vi "Get_Next_Sub_Collection.vi"(8 "error in (no error)":errorcluster caption="entrée d'erreur (pas d'erreur)", 11 "Firebase Packaging en entrée":refnum<class "Firebase Packaging.lvclass">) -> (0 "error out":errorcluster caption="sortie d'erreur", 3 "Firebase Packaging en sortie":refnum<class "Firebase Packaging.lvclass">)   [LabVIEW 2020, in "Library Instrument & Equipement.lvlib" / "Library FireBase.lvlib" / "Firebase Packaging.lvclass"]
doc: "Return the documents present in the test collection for each DATA read with Get_Data\nPlease initialise the following values\n - Name BDD\n - Document of test sequence\n - API Key\n - Nb To Read"
uses:
  Firebase Packaging.lvclass
  C:/Users/ngarcin/OneDrive - Altyor/Standard TB/Class/Firebase/Source/Firebase Driver/Firebase Driver.lvclass
  Firebase Packaging.lvclass/Firebase Packaging.ctl
  JSON API/JSON Value/JSON Value.lvclass
  JSON API/JSON Value/Set from JSON string.vi
  Firebase Altyor/Firebase Altyor.lvclass
  JSON API/Variant JSON/Variant JSON.lvlib
  JSON API/Get Polymorphic/JSON GetSet.lvlib
  Firebase Driver/Firebase Driver.lvclass
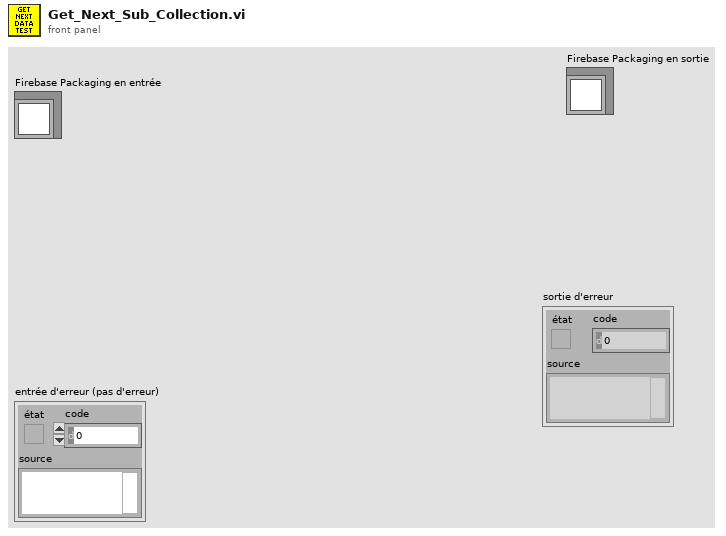
[diagram p1: front panel]
types:
  T1 = cluster{"documents":cluster{"name":string, "fields":cluster{"Result":cluster{"booleanValue":bool}, "CreationDate":cluster{"timestampValue":string}, "Batch":cluster{"stringValue":string}, "SerialNumber":cluster{"stringValue":string}, "EndOfProduction":cluster{"timestampValue":string}, "PartNumber":cluster{"stringValue":string}, "OrderNumber":cluster{"stringValue":string}, "Operator":cluster{"stringValue":string}}}[]}
  T2 = cluster{"name":string, "fields":cluster{"SN_Produit":cluster{"stringValue":string}, "Product_Name":cluster{"stringValue":string}}}[][]
  T3 = cluster{"name":string, "fields":cluster{"Result":cluster{"booleanValue":bool}, "CreationDate":cluster{"timestampValue":string}, "Batch":cluster{"stringValue":string}, "SerialNumber":cluster{"stringValue":string}, "EndOfProduction":cluster{"timestampValue":string}, "PartNumber":cluster{"stringValue":string}, "OrderNumber":cluster{"stringValue":string}, "Operator":cluster{"stringValue":string}}}[]
  T4 = cluster{"name":string, "fields":cluster{"SN_Produit":cluster{"stringValue":string}, "Product_Name":cluster{"stringValue":string}}}[]
  T5 = cluster{"documents":cluster{"name":string, "fields":cluster{"SN_Produit":cluster{"stringValue":string}, "Product_Name":cluster{"stringValue":string}}}[], "nextPageToken":string}
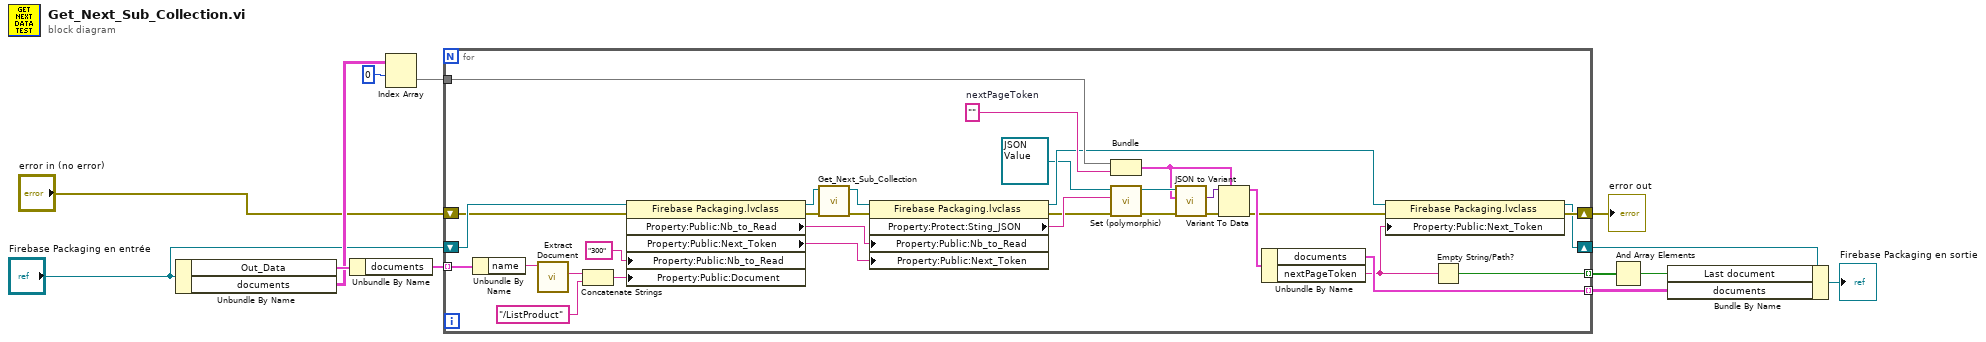
[diagram p0: block diagram]
diagram:
  n1 = Unbundle By Name("Firebase Packaging en entrée") -> ("Out_Data"=w13:T1, "documents"=w10:T2)
  n2 = Unbundle By Name(w13) -> ("documents"=w12:T3)
  n3 = Index Array(array=w10, index (row)=0 ("indice (ligne)")) -> (element=w9:T4)  [unwired: 1 in]
  n4 = for {
    tunnel: [w21] -> w11 mode=indexing
    shift-right: [w23] -> w7
    shift-left: "Firebase Packaging en entrée" -> [w38]
    shift-right: [w25] -> w3
    shift-left: "error in (no error)" -> [w37]
    tunnel: w12 -> [w36] mode=indexing
    tunnel: w9 -> [w28]
    tunnel: [w14] -> w2 mode=indexing
    w40 = ""  # nextPageToken
    n5 = Unbundle By Name(w36) -> ("name"=w35:string)
    n6 = call "Extract Document.vi"("Name"=w35) -> ("Source"=w34:string)  [unwired: 9 in, 1 out]
    n7 = Concatenate Strings(w34, "/ListProduct" ("chaîne")) -> (w32:string)
    n8 = property class="Firebase Packaging.lvclass"(reference=w38, error in=w37, "Property:Public:Nb_to_Read"="300" ("Nb_to_Read"), "Property:Public:Document"=w32) -> (reference out=w16:refnum<class "Firebase Packaging.lvclass">, error out=w19:errorcluster, "Property:Public:Nb_to_Read"=w31:string, "Property:Public:Next_Token"=w29:string)
    n9 = call-parent "Get_Next_Sub_Collection.vi"("error in (no error)"=w19, "Firebase Altyor en entrée"=w16) -> ("error out"=w18:errorcluster, "Firebase Altyor en sortie"=w17:refnum<class "Firebase Packaging.lvclass">)  [unwired: 8 in]
    n10 = property class="Firebase Packaging.lvclass"(reference=w17, error in=w18, "Property:Public:Nb_to_Read"=w31, "Property:Public:Next_Token"=w29) -> (reference out=w24:refnum<class "Firebase Packaging.lvclass">, error out=w27:errorcluster, "Property:Protect:Sting_JSON"=w42:string)
    n11 = Bundle("documents"=w28, "nextPageToken"=w40) -> (w39:T5)  [unwired: 1 in]
    n12 = call-poly "Set (polymorphic).vi"("error in (no error)"=w27, "JSON stream"=w42, "JSON Value in"=refnum<class "JSON Value.lvclass"> refnum) -> ("error out"=w43:errorcluster, "JSON Value out"=w45:refnum<class "JSON Value.lvclass">)  [unwired: 6 in, 1 out]
    n13 = call "JSON to Variant.vi"("error in (no error)"=w43, "Variant (Data Type)"=w39, "JSON Value"=w45) -> ("error out"=w44:errorcluster, "Variant out"=w20:variant)  [unwired: 7 in]
    n14 = Variant To Data(error in=w44, type=w39, Variant=w20) -> (data=w41:T5, error out=w26:errorcluster)
    n15 = Unbundle By Name(w41) -> ("documents"=w21:T4, "nextPageToken"=w15:string)
    n16 = property class="Firebase Packaging.lvclass"(reference=w24, error in=w26, "Property:Public:Next_Token"=w15) -> (reference out=w23:refnum<class "Firebase Packaging.lvclass">, error out=w25:errorcluster)
    n17 = Empty String/Path?(string/path=w15) -> (empty?=w14:bool)
  }
  "error out" <- w3
  n18 = And Array Elements(Boolean array=w2) -> (logical AND=w1:bool)
  n19 = Bundle By Name(cluster=w7, "Last document"=w1, "documents"=w11) -> (→"Firebase Packaging en sortie":refnum<class "Firebase Packaging.lvclass">)
